vi "Z_state_VCH.vi"(9 "Time":u32[](array[numeric])=[1000, 10000], 10 "Alarm":bool[](array[boolean])=[FALSE, FALSE], 11 "Z_In":T4={"Z_Source"=enum."local disabled", "Z_State"=enum."initialization", "ZM_State"=enum."initialization"}) -> (1 "t":u32, 3 "Z_Out":T4={"Z_Source"=enum."local disabled", "Z_State"=enum."initialization", "ZM_State"=enum."initialization"})   [LabVIEW 2019, in "Valves.lvlib"]
uses:
  Valves.lvlib
  Heating/ctl/Y_source.ctl
  ctl/Z_State_VCH.ctl
  ctl/ZM_State_VCH.ctl
  Trigers/RS.vi
  Timer Delay/Timer.vi
  Userlib.lvlib
  Heating/Heating.lvlib
panel:
  # "Alarm_L1"
  # "Alarm_L2"
  # "TsStop"
  # "T_check"
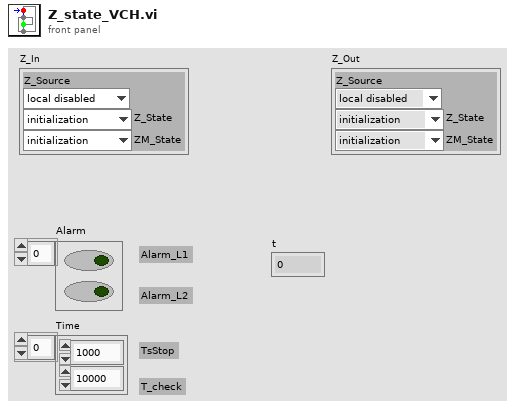
[diagram p1: front panel]
types:
  T1 = typedef "Heating.lvlib/Y_source.ctl" = enum8{"initialize", "local disabled", "local hand", "hand", "auto", "dist"}
  T2 = typedef "Valves.lvlib/Z_State_VCH.ctl" = enum8{"initialization", "alarm", "disabled", "not ready", "closed ready", "reserv", "reserv1", "reserv2", "reserv3", "check", "on min", "open", "on (closed)"}
  T3 = typedef "Valves.lvlib/ZM_State_VCH.ctl" = enum8{"initialization", "closed", "big_pause", "little_pause", "open", "close_cmd"}
  T4 = cluster{"Z_Source":T1, "Z_State":T2, "ZM_State":T3}
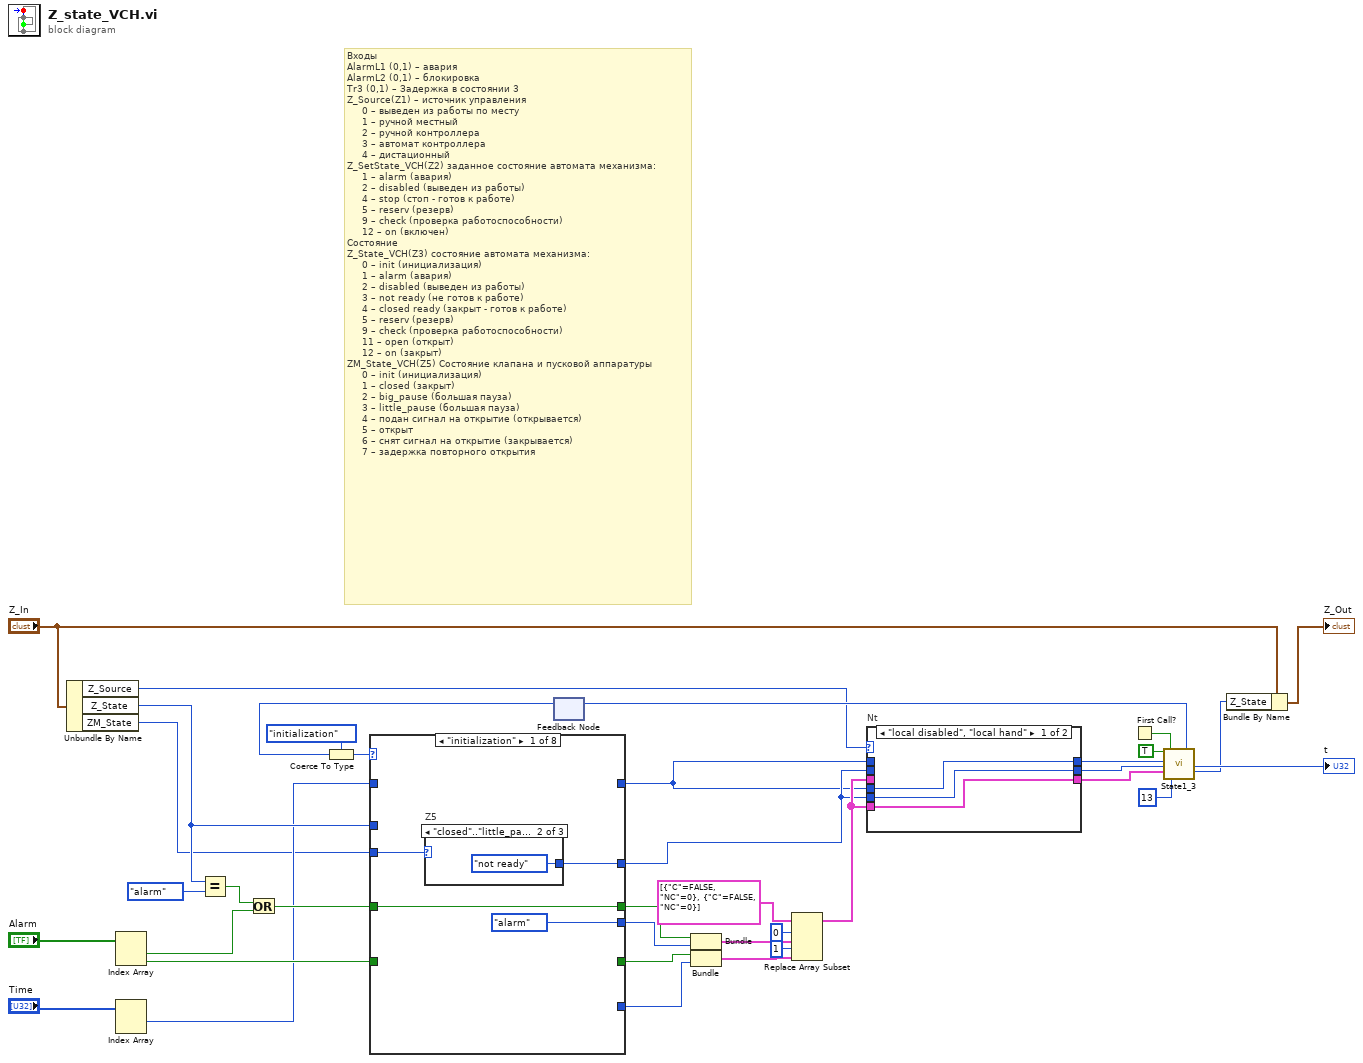
[diagram p0: block diagram]
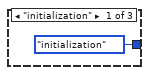
[diagram p3: hidden frame]
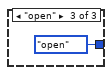
[diagram p4: hidden frame]
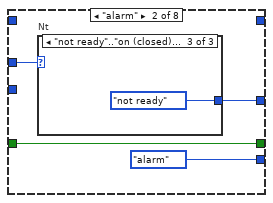
[diagram p5: hidden frame]
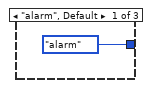
[diagram p6: hidden frame]
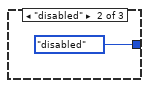
[diagram p7: hidden frame]
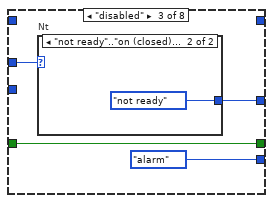
[diagram p8: hidden frame]
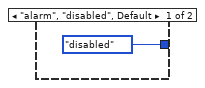
[diagram p9: hidden frame]
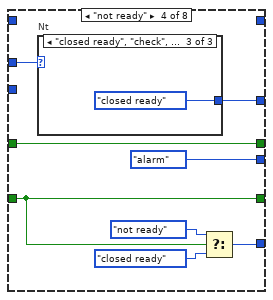
[diagram p10: hidden frame]
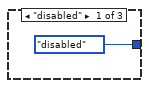
[diagram p11: hidden frame]
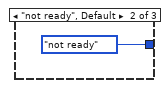
[diagram p12: hidden frame]
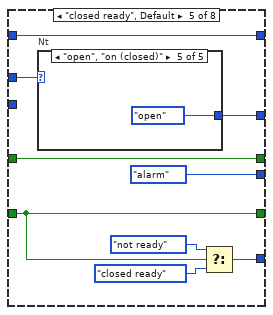
[diagram p13: hidden frame]
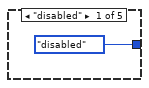
[diagram p14: hidden frame]
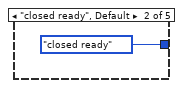
[diagram p15: hidden frame]
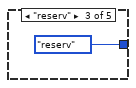
[diagram p16: hidden frame]
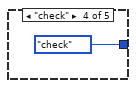
[diagram p17: hidden frame]
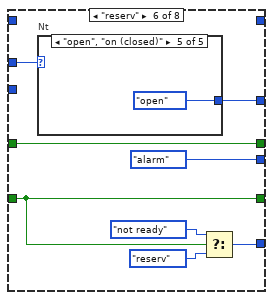
[diagram p18: hidden frame]
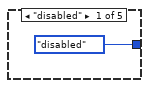
[diagram p19: hidden frame]
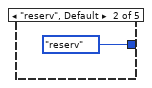
[diagram p20: hidden frame]
diagram:
  # "Входы\nAlarmL1 (0,1) – авария\nAlarmL2 (0,1) – блокировка\nTr3 (0,1) – Задержка в состоянии 3\nZ_Source(Z1) – источник управления\n     0 – выведен из работы по месту\n     1 – ручной местный\n     2 – ручной контроллера\n     3 – автомат контроллера\n     4 – дистационный\nZ_SetState_VCH(Z2) заданное состояние автомата механизма:\n     1 – alarm (авария)\n     2 – disabled (выведен из работы)\n     4 – stop (стоп - готов к работе)\n     5 – reserv (резерв)\n     9 – check (проверка работоспособности)\n     12 – on (включен)\nСостояние\nZ_State_VCH(Z3) состояние автомата механизма:\n     0 – init (инициализация)\n     1 – alarm (авария)\n     2 – disabled (выведен из работы)\n     3 – not ready (не готов к работе)\n     4 – closed ready (закрыт - готов к работе)\n     5 – reserv (резерв)\n     9 – check (проверка работоспособности)\n     11 – open (открыт)\n     12 – on (закрыт)\nZM_State_VCH(Z5) Состояние клапана и пусковой аппаратуры\n     0 – init (инициализация)\n     1 – сlosed (закрыт)\n     2 – big_pause (большая пауза)\n     3 – little_pause (большая пауза)\n     4 – подан сигнал на открытие (открывается)\n     5 – открыт\n     6 – снят сигнал на открытие (закрывается)\n     7 – задержка повторного открытия"
  n1 = Unbundle By Name("Z_In") -> ("Z_Source"=w16:T1, "Z_State"=w14:T2, "ZM_State"=w6:T3)
  n2 = Index Array(array="Alarm") -> (element #1=w9:bool, element #2=w8:bool)  [unwired: 2 in]
  n3 = Index Array(array="Time") -> (element #1=w7:u32)  [unwired: 2 in, 1 out]
  n4 = Equal?(x=w14, y=Z_State_VCH."alarm" ("Z_State")) -> (x = y?=w37:bool)
  n5 = Or(x=w37, y=w9) -> (x .or. y?=w36:bool)
  n6 = feedback #1() -> (w33:u32)  [unwired: 1 in]
  n7 = Coerce To Type(0:w33, 1:Z_State_VCH."initialization" ("X5(DistSetSate) 2")) -> (2:w34:T2)
  n8 = case shown="\"initialization\"" w34 {
    tunnel: w36 -> [w41 w48 w55 w59 w77 w90 w103 w130]
    tunnel: w8 -> [_ _ _ w58 w71 w84 w99 w125]
    tunnel: w6 -> [w38 _ _ _ _ _ w98 w126]
    tunnel: w7 -> [_ _ _ _ w69 _ _ _]
    tunnel: [w41 w48 w55 w59 w77 w90 w103 w130] -> w23
    tunnel: [Z_State_VCH."alarm" ("state next") Z_State_VCH."alarm" ("state next") Z_State_VCH."alarm" ("state next") Z_State_VCH."alarm" ("state next") Z_State_VCH."alarm" ("state next") Z_State_VCH."alarm" ("state next") Z_State_VCH."alarm" ("state next") Z_State_VCH."alarm" ("state next")] -> w22
    tunnel: [w39 w47 w54 w64 w75 w88 w101 w128] -> w3
    tunnel: [_ _ _ w60 w70 w83 w96 Z_State_VCH."not ready" ("state next")] -> w20
    tunnel: [_ _ _ w58 w71 w84 w97 w125] -> w21
    tunnel: [_ _ _ _ w69 _ _ _] -> w1
    tunnel: w14 -> [_ w46 w53 w65 w76 w89 w102 w129]
    frame "initialization" {
      n9 = case "Z5" shown="\"closed\"..\"little_pause\", Default" w38 {
        tunnel: [Z_State_VCH."initialization" ("state next") Z_State_VCH."not ready" ("state next") Z_State_VCH."open" ("state next")] -> w39
        frame "initialization" {
        }
        frame "closed".."little_pause", Default {
        }
        frame "open" {
        }
      }
    }
    frame "alarm" {
      n10 = case "Nt" shown="\"not ready\"..\"on (closed)\"" w46 {
        tunnel: [Z_State_VCH."alarm" ("state next") Z_State_VCH."disabled" ("state next") Z_State_VCH."not ready" ("state next")] -> w47
        frame "alarm", Default {
        }
        frame "disabled" {
        }
        frame "not ready".."on (closed)" {
        }
      }
    }
    frame "disabled" {
      n11 = case "Nt" shown="\"not ready\"..\"on (closed)\"" w53 {
        tunnel: [Z_State_VCH."disabled" ("state next") Z_State_VCH."not ready" ("state next")] -> w54
        frame "alarm", "disabled", Default {
        }
        frame "not ready".."on (closed)" {
        }
      }
    }
    frame "not ready" {
      n12 = case "Nt" shown="\"closed ready\", \"check\", \"open\", \"on (closed)\"" w65 {
        tunnel: [Z_State_VCH."disabled" ("state next") Z_State_VCH."not ready" ("state next") Z_State_VCH."closed ready" ("state next")] -> w64
        frame "disabled" {
        }
        frame "not ready", Default {
        }
        frame "closed ready", "check", "open", "on (closed)" {
        }
      }
      n13 = Select(t=Z_State_VCH."not ready" ("state next"), s=w58, f=Z_State_VCH."closed ready" ("state next")) -> (s? t:f=w60:T2)
    }
    frame "closed ready", Default {
      n14 = case "Nt" shown="\"open\", \"on (closed)\"" w76 {
        tunnel: [Z_State_VCH."disabled" ("state next") Z_State_VCH."closed ready" ("state next") Z_State_VCH."reserv" ("state next") Z_State_VCH."check" ("state next") Z_State_VCH."open" ("state next")] -> w75
        frame "disabled" {
        }
        frame "closed ready", Default {
        }
        frame "reserv" {
        }
        frame "check" {
        }
        frame "open", "on (closed)" {
        }
      }
      n15 = Select(t=Z_State_VCH."not ready" ("state next"), s=w71, f=Z_State_VCH."closed ready" ("state next")) -> (s? t:f=w70:T2)
    }
    frame "reserv" {
      n16 = case "Nt" shown="\"open\", \"on (closed)\"" w89 {
        tunnel: [Z_State_VCH."disabled" ("state next") Z_State_VCH."reserv" ("state next") Z_State_VCH."closed ready" ("state next") Z_State_VCH."check" ("state next") Z_State_VCH."open" ("state next")] -> w88
        frame "disabled" {
        }
        frame "reserv", Default {
        }
        frame "closed ready" {
        }
        frame "check" {
        }
        frame "open", "on (closed)" {
        }
      }
      n17 = Select(t=Z_State_VCH."not ready" ("state next"), s=w84, f=Z_State_VCH."reserv" ("state next")) -> (s? t:f=w83:T2)
    }
    frame "check" {
      n18 = case "Nt" shown="\"disabled\"" w102 {
        tunnel: [w111 w115 Z_State_VCH."check" ("state next") w120] -> w101
        tunnel: w98 -> [w112 w116 _ w121]
        frame "disabled" {
          n19 = case "Z5" shown="\"closed\"..\"little_pause\", Default" w112 {
            tunnel: [Z_State_VCH."disabled" ("state next") Z_State_VCH."check" ("state next")] -> w111
            frame "closed".."little_pause", Default {
            }
            frame "open", "close_cmd" {
            }
          }
        }
        frame "closed ready", "reserv", Default {
          n20 = case "Z5" shown="\"closed\"..\"little_pause\", Default" w116 {
            tunnel: [Z_State_VCH."closed ready" ("state next") Z_State_VCH."check" ("state next")] -> w115
            frame "closed".."little_pause", Default {
            }
            frame "open", "close_cmd" {
            }
          }
        }
        frame "check" {
        }
        frame "open", "on (closed)" {
          n21 = case "Z5" shown="\"closed\"..\"little_pause\", Default" w121 {
            tunnel: [Z_State_VCH."on (closed)" ("state next") Z_State_VCH."open" ("state next")] -> w120
            frame "closed".."little_pause", Default {
            }
            frame "open" {
            }
          }
        }
      }
      n22 = case "Nt" shown="True" w99 {
        selector: w99 -> [w104 w109]
        tunnel: [w105 Z_State_VCH."check" ("state next")] -> w96
        tunnel: w98 -> [w106 _]
        tunnel: [w104 w109] -> w97
        frame True {
          n23 = case "Z5" shown="\"closed\"..\"little_pause\", Default" w106 {
            tunnel: [Z_State_VCH."not ready" ("state next") Z_State_VCH."check" ("state next")] -> w105
            frame "closed".."little_pause", Default {
            }
            frame "open", "close_cmd" {
            }
          }
        }
        frame False {
        }
      }
    }
    frame "open", "on (closed)" {
      n24 = case "Nt" shown="\"closed ready\", \"reserv\", Default" w129 {
        tunnel: [w131 w135 w139] -> w128
        tunnel: w126 -> [w132 w136 w140]
        frame "disabled" {
          n25 = case "Z5" shown="\"closed\"..\"little_pause\", Default" w132 {
            tunnel: [Z_State_VCH."disabled" ("state next") Z_State_VCH."open" ("state next")] -> w131
            frame "closed".."little_pause", Default {
            }
            frame "open", "close_cmd" {
            }
          }
        }
        frame "closed ready", "reserv", Default {
          n26 = case "Z5" shown="\"closed\"..\"little_pause\", Default" w136 {
            tunnel: [Z_State_VCH."closed ready" ("state next") Z_State_VCH."open" ("state next")] -> w135
            frame "closed".."little_pause", Default {
            }
            frame "open", "close_cmd" {
            }
          }
        }
        frame "open", "on (closed)" {
          n27 = case "Z5" shown="\"closed\"..\"little_pause\", Default" w140 {
            tunnel: [Z_State_VCH."on (closed)" ("state next") Z_State_VCH."open" ("state next")] -> w139
            frame "closed".."little_pause", Default {
            }
            frame "open", "close_cmd" {
            }
          }
        }
      }
    }
  }
  n28 = Bundle(w23, "state next"=w22) -> (w26:cluster{bool, "state next":T2})  [unwired: 1 in]
  n29 = Bundle("Alarm"=w21, "state next"=w20) -> (w24:cluster{"Alarm":bool, "state next":T2})  [unwired: 1 in]
  n30 = Replace Array Subset(array=cluster{"C":bool, "NC":u32}[] [{"C"=FALSE, "NC"=0}, {"C"=FALSE, "NC"=0}] ("appended array"), new element #1=w26, index #1=0 ("index"), new element #2=w24, index #2=1 ("index")) -> (w12:cluster{"C":bool, "NC":u32}[])
  n31 = case "Nt" shown="\"local disabled\", \"local hand\"" w16 {
    tunnel: w3 -> [_ w148]
    tunnel: w12 -> [_ w147]
    tunnel: [w144 w148] -> w18
    tunnel: [w145 w147] -> w17
    tunnel: w3 -> [w144 _]
    tunnel: w12 -> [w145 _]
    tunnel: w1 -> [_ w146]
    tunnel: [w143 w146] -> w2
    tunnel: w1 -> [w143 _]
    frame "local disabled", "local hand" {
    }
    frame "hand".."dist", Default {
    }
  }
  n32 = First Call?() -> (First Call?: T/F=w31:bool)
  n33 = call "State1_3.vi"("Start"=TRUE, "t"=w2, "Nt"=w18, "C_table"=w17, "Reset"=w31, "End step"=u32 13) -> ("N next"=w29:u32, "t"=→"t":u32, "N curr"=w15:u32)  [unwired: 8 in, 3 out]
  n34 = feedback-in #1(w29) -> ()
  n35 = Bundle By Name(cluster="Z_In", "Z_State"=w15) -> (→"Z_Out":T4)
